vi "Network Stream.vi"() -> ()   [LabVIEW 2014]
doc: "In this demo we cover network streams. Pretty similar to the camera stream demo, the stream is opened and continuously grabs images from the stream.\n\nThe default value for the network address is a online published stream.\n\n<b>Disclaimer:</b>\nAny links to external websites and/or non-MSC information provided by this library are provided as a courtesy. They should not be construed as an endorsement by MSC of the content or views of the linked materials. We have no control over the nature, content and availability of those sites and you view them strictly at your own risk."
uses:
  MSC Video_class/MSC Video.lvclass
  MSC Image_class/MSC Image.lvclass
panel:
  in  "Network Address":string="http://devimages.apple.com/iphone/samples/bipbop/gear1/prog_index.m3u8"
  out "error out":errorcluster
  in  "stop":bool
  out "Live Image":picture
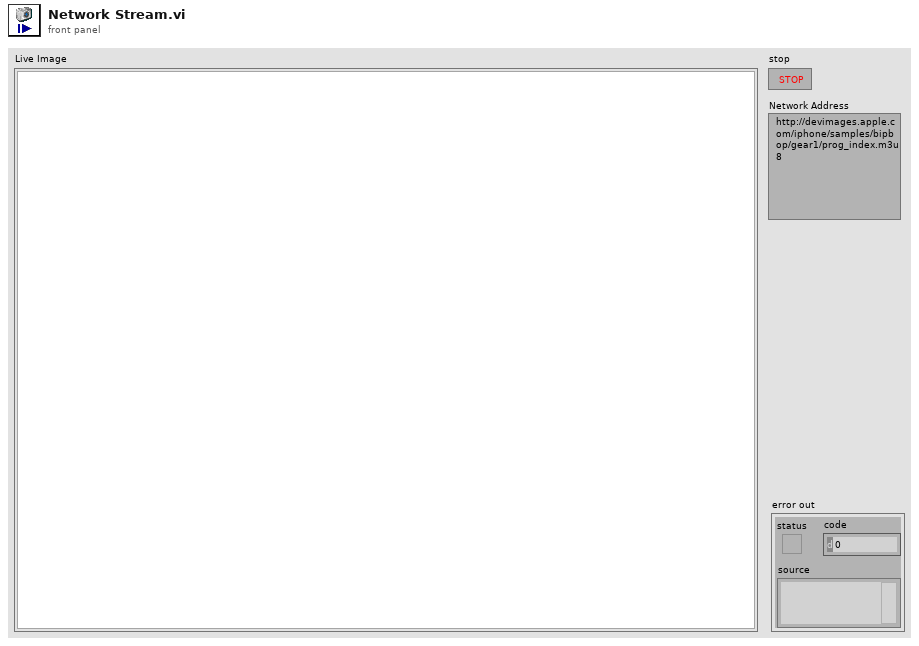
[diagram p1: front panel]
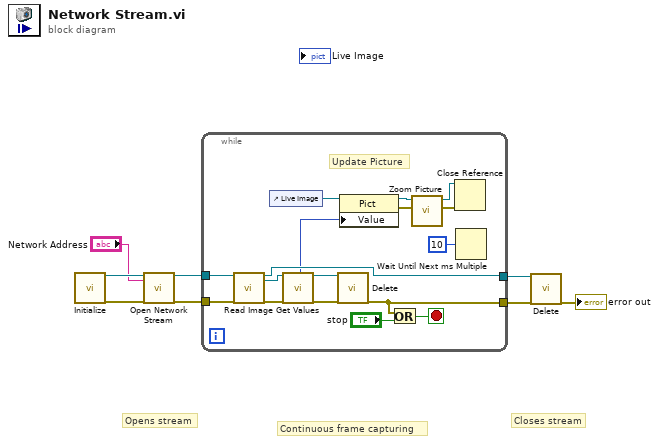
[diagram p0: block diagram]
diagram:
  # "Closes stream"
  # "Continuous frame capturing"
  # "Opens stream"
  n1 = call "Initialize.vi"() -> ("video out"=w4:refnum<class "MSC Video.lvclass">, "error out"=w5:errorcluster)  [unwired: 18 in]
  n2 = call-dynamic "Open Network Stream.vi"("video in"=w4, "Network Address"="Network Address", "error in (no error)"=w5) -> ("video out"=w3:refnum<class "MSC Video.lvclass">, "error out"=w2:errorcluster)  [unwired: 15 in]
  n3 = while {
    tunnel: w3 -> [w25]
    tunnel: w2 -> [w24]
    tunnel: [w22] -> w8
    tunnel: [w16] -> w7
    stop <- w23 stop-if-true
    # "Update Picture"
    n4 = call-dynamic "Read Image.vi"("video in"=w25, "error in (no error)"=w24) -> ("video out"=w22:refnum<class "MSC Video.lvclass">, "image out"=w21:refnum<class "MSC Image.lvclass">, "error out"=w20:errorcluster)  [unwired: 15 in]
    n5 = control-ref of="Live Image"() -> (w15:refnum<vi>)
    n6 = call-dynamic "Get Values.vi"("image in"=w21, "error in (no error)"=w20) -> ("picture"=w10:picture, "image out"=w18:refnum<class "MSC Image.lvclass">, "error out"=w17:errorcluster)  [unwired: 10 in, 5 out]
    n7 = call-dynamic "Delete.vi"("image in"=w18, "error in (no error)"=w17) -> ("error out"=w16:errorcluster)  [unwired: 17 in]
    n8 = property class="Pict"(reference=w15, "Value"=w10) -> (reference out=w11:refnum<vi>, error out=w12:errorcluster)  [unwired: 1 in]
    n9 = Or(x=w16, y="stop") -> (x .or. y?=w23:bool)
    n10 = call "Zoom Picture.vi"("error in (no error)"=w12, "Picture in"=w11) -> ("error out"=w14:errorcluster, "Picture out"=w13:refnum<vi>)  [unwired: 8 in]
    n11 = Close Reference(reference=w13, error in (no error)=w14) -> ()  [unwired: 1 out]
    n12 = Wait Until Next ms Multiple(millisecond multiple=u32 10) -> ()  [unwired: 1 out]
  }
  n13 = call-dynamic "Delete.vi"("video in"=w8, "error in (no error)"=w7) -> ("error out"=→"error out":errorcluster)  [unwired: 17 in]
